vi "OP100 Indicators.vi"(8 "error in (no error)":errorcluster, 10 "Array":refnum<vi>[](array[refnum]), 11 "OUTPUT INDICATOR":T1={"OP - 10"={"BARCODE"="", "LEAK RATE"=0.0, "RESULT"=FALSE}, "OP - 30"={"BARCODE"="", "Displacement"=0.0, "Load"=0.0, "Middle Gear Shaft Status"=FALSE, "Final Result"=FALSE}, "OP - 60"={"BARCODE"="", "Screw 1 Data"=0.0, "Screw 2 data"=0.0, "Screw 1 Status"=FALSE, "Screw 2 Status"=FALSE, "Screw3 Data"=0.0, "Final Result"=FALSE, "Screw3 Status"=FALSE, "Screw4 Data"=0.0, "Screw5 Data"=0.0, "Screw4 Status"=FALSE, "Screw5 Status"=FALSE, "Screw6 Data"=0.0, "Screw6 Status"=FALSE}, "OP - 70"={"BARCODE"="", "Sensor MIN Vltg"=0.0, "Sensor MAX Vltg"=0.0, "Final Result"=FALSE}, "OP - 80"={"BARCODE"="", "Load"=0.0, "Final Result"=FALSE, "Dispensing"=FALSE}, "OP - 90"={"BARCODE"="", "Seat LT Data"=0.0, "Seat Status"=FALSE, "Steam LT Data"=0.0, "Final Result"=FALSE}, "OP - 110"={"BARCODE"=""}, "OP - 20"={"BARCODE"="", "Bottom Displace"=0.0, "Bottom Load"=0.0, "Camera Status"=FALSE, "Bottom Result"=TRUE, "Top Displace"=0.0, "Top Load "=0.0, "Camera Status"=FALSE, "Top Result"=FALSE, "Final Result"=FALSE}, "OP - 40"={"BARCODE"="", "RH Screw"=0.0, "LH Screw "=0.0, "RH Status"=FALSE, "LH Status"=FALSE, "Dispalcement "=0.0, "Stack Load "=0.0, "Final Result"=FALSE}, "OP - 50"={"BARCODE"="", "Nut Torque"=0.0, "LH Motor Screw"=0.0, "LH Status"=FALSE, "RH Status"=FALSE, "RH Motor Screw"=0.0, "Final Result"=FALSE, "Nut Status"=FALSE, "Camera Status"=FALSE}, "OP - 100"={"BARCODE"="", "Sensor O/P Open"=0.0, "Sensor O/P Start Of Close"=0.0, "Final Result"=FALSE, "Sensor O/P Full Close"=0.0, "Motor Peak"=0.0, "Motor Start Of Close"=0.0, "Motor Full Close"=0.0, "Motor Start Back"=0.0, "Motor Full Open"=0.0, "Response time FWD"=0.0, "Response Time REV"=0.0}}) -> (0 "error out":errorcluster, 3 "OUTPUT INDICATOR":T1={"OP - 10"={"BARCODE"="", "LEAK RATE"=0.0, "RESULT"=FALSE}, "OP - 30"={"BARCODE"="", "Displacement"=0.0, "Load"=0.0, "Middle Gear Shaft Status"=FALSE, "Final Result"=FALSE}, "OP - 60"={"BARCODE"="", "Screw 1 Data"=0.0, "Screw 2 data"=0.0, "Screw 1 Status"=FALSE, "Screw 2 Status"=FALSE, "Screw3 Data"=0.0, "Final Result"=FALSE, "Screw3 Status"=FALSE, "Screw4 Data"=0.0, "Screw5 Data"=0.0, "Screw4 Status"=FALSE, "Screw5 Status"=FALSE, "Screw6 Data"=0.0, "Screw6 Status"=FALSE}, "OP - 70"={"BARCODE"="", "Sensor MIN Vltg"=0.0, "Sensor MAX Vltg"=0.0, "Final Result"=FALSE}, "OP - 80"={"BARCODE"="", "Load"=0.0, "Final Result"=FALSE, "Dispensing"=FALSE}, "OP - 90"={"BARCODE"="", "Seat LT Data"=0.0, "Seat Status"=FALSE, "Steam LT Data"=0.0, "Final Result"=FALSE}, "OP - 110"={"BARCODE"=""}, "OP - 20"={"BARCODE"="", "Bottom Displace"=0.0, "Bottom Load"=0.0, "Camera Status"=FALSE, "Bottom Result"=TRUE, "Top Displace"=0.0, "Top Load "=0.0, "Camera Status"=FALSE, "Top Result"=FALSE, "Final Result"=FALSE}, "OP - 40"={"BARCODE"="", "RH Screw"=0.0, "LH Screw "=0.0, "RH Status"=FALSE, "LH Status"=FALSE, "Dispalcement "=0.0, "Stack Load "=0.0, "Final Result"=FALSE}, "OP - 50"={"BARCODE"="", "Nut Torque"=0.0, "LH Motor Screw"=0.0, "LH Status"=FALSE, "RH Status"=FALSE, "RH Motor Screw"=0.0, "Final Result"=FALSE, "Nut Status"=FALSE, "Camera Status"=FALSE}, "OP - 100"={"BARCODE"="", "Sensor O/P Open"=0.0, "Sensor O/P Start Of Close"=0.0, "Final Result"=FALSE, "Sensor O/P Full Close"=0.0, "Motor Peak"=0.0, "Motor Start Of Close"=0.0, "Motor Full Close"=0.0, "Motor Start Back"=0.0, "Motor Full Open"=0.0, "Response time FWD"=0.0, "Response Time REV"=0.0}})   [LabVIEW 2017]
uses:
  2f4ed2d2-b3e5-497f-b08f-b9010f661fe3.vi
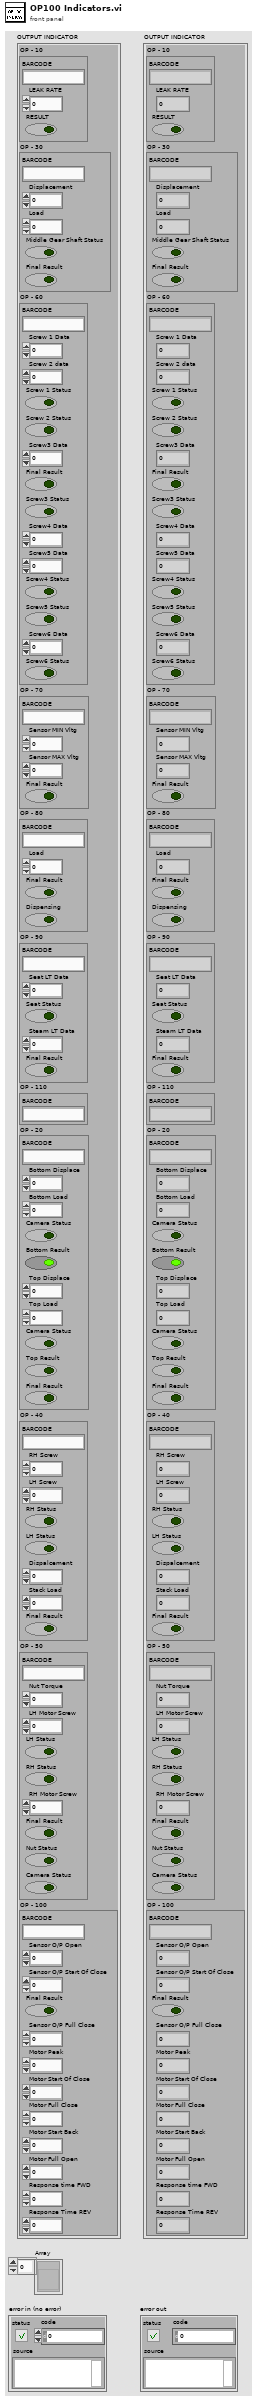
[diagram p1: front panel]
types:
  T1 = cluster{"OP - 10":cluster{"BARCODE":string, "LEAK RATE":dbl, "RESULT":bool}, "OP - 30":cluster{"BARCODE":string, "Displacement":dbl, "Load":dbl, "Middle Gear Shaft Status":bool, "Final Result":bool}, "OP - 60":cluster{"BARCODE":string, "Screw 1 Data":dbl, "Screw 2 data":dbl, "Screw 1 Status":bool, "Screw 2 Status":bool, "Screw3 Data":dbl, "Final Result":bool, "Screw3 Status":bool, "Screw4 Data":dbl, "Screw5 Data":dbl, "Screw4 Status":bool, "Screw5 Status":bool, "Screw6 Data":dbl, "Screw6 Status":bool}, "OP - 70":cluster{"BARCODE":string, "Sensor MIN Vltg":dbl, "Sensor MAX Vltg":dbl, "Final Result":bool}, "OP - 80":cluster{"BARCODE":string, "Load":dbl, "Final Result":bool, "Dispensing":bool}, "OP - 90":cluster{"BARCODE":string, "Seat LT Data":dbl, "Seat Status":bool, "Steam LT Data":dbl, "Final Result":bool}, "OP - 110":cluster{"BARCODE":string}, "OP - 20":cluster{"BARCODE":string, "Bottom Displace":dbl, "Bottom Load":dbl, "Camera Status":bool, "Bottom Result":bool, "Top Displace":dbl, "Top Load ":dbl, "Camera Status":bool, "Top Result":bool, "Final Result":bool}, "OP - 40":cluster{"BARCODE":string, "RH Screw":dbl, "LH Screw ":dbl, "RH Status":bool, "LH Status":bool, "Dispalcement ":dbl, "Stack Load ":dbl, "Final Result":bool}, "OP - 50":cluster{"BARCODE":string, "Nut Torque":dbl, "LH Motor Screw":dbl, "LH Status":bool, "RH Status":bool, "RH Motor Screw":dbl, "Final Result":bool, "Nut Status":bool, "Camera Status":bool}, "OP - 100":cluster{"BARCODE":string, "Sensor O/P Open":dbl, "Sensor O/P Start Of Close":dbl, "Final Result":bool, "Sensor O/P Full Close":dbl, "Motor Peak":dbl, "Motor Start Of Close":dbl, "Motor Full Close":dbl, "Motor Start Back":dbl, "Motor Full Open":dbl, "Response time FWD":dbl, "Response Time REV":dbl}}
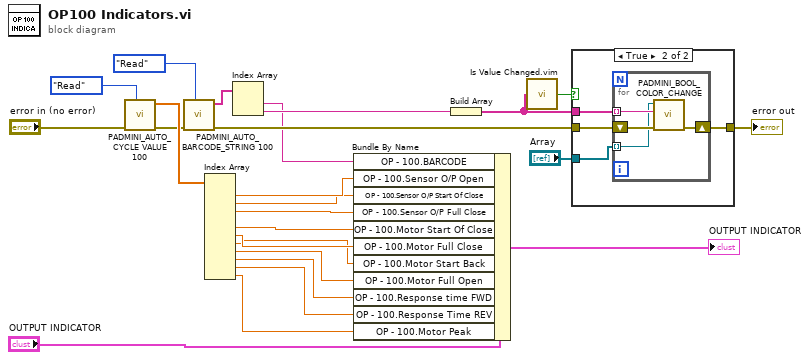
[diagram p0: block diagram]
diagram:
  n1 = call "PADMINI_AUTO_CYCLE VALUE 100.vi"("Enum"=enum16{"Read", "Write"}."Read", "error in (no error)"="error in (no error)") -> ("error out"=w18:errorcluster, "Input 2"=w21:sgl[])  [unwired: 8 in]
  n2 = call "PADMINI_AUTO_BARCODE_STRING 100.vi"("Enum"=enum16{"Read", "Write"}."Read", "error in (no error)"=w18) -> ("error out"=w19:errorcluster, "Input 2"=w24:string[])  [unwired: 8 in]
  n3 = Index Array(array=w21) -> (element #1=w10:sgl, element #2=w9:sgl, element #3=w8:sgl, element #5=w7:sgl, element #6=w6:sgl, element #7=w5:sgl, element #8=w4:sgl, element #9=w3:sgl, element #10=w2:sgl, element #11=w1:sgl)  [unwired: 11 in, 1 out]
  n4 = Index Array(array=w24) -> (element #1=w11:string, element #2=w13:string)  [unwired: 2 in]
  n5 = Bundle By Name(cluster="OUTPUT INDICATOR", "OP - 100.BARCODE"=w11, "OP - 100.Sensor O/P Open"=w10, "OP - 100.Sensor O/P Start Of Close"=w9, "OP - 100.Sensor O/P Full Close"=w8, "OP - 100.Motor Start Of Close"=w7, "OP - 100.Motor Full Close"=w6, "OP - 100.Motor Start Back"=w5, "OP - 100.Motor Full Open"=w4, "OP - 100.Response time FWD"=w3, "OP - 100.Response Time REV"=w2, "OP - 100.Motor Peak"=w1) -> (→"OUTPUT INDICATOR":T1)
  n6 = Build Array(w13) -> (w14:string[])
  n7 = call "Is Value Changed.vim"("value"=w14) -> ("changed or first call?"=w12:bool)
  n8 = case shown="True" w12 {
    tunnel: [w26 w30] -> w20
    tunnel: w14 -> [_ w29]
    tunnel: w19 -> [w26 w28]
    tunnel: "Array" -> [_ w27]
    frame False {
    }
    frame True {
      n9 = for {
        tunnel: w29 -> [w33] mode=indexing
        shift-right: [w34] -> w30
        shift-left: w28 -> [w32]
        tunnel: w27 -> [w31] mode=indexing
        n10 = call "PADMINI_BOOL_COLOR_CHANGE.vi"("error in (no error)"=w32, "Input Result"=w33, "Boolean in"=w31) -> ("error out"=w34:errorcluster)  [unwired: 8 in]
      }
    }
  }
  "error out" <- w20
